vi "attribute_Express_SubVI.vi"(0 "VISA resource name":refnum<visa-resource-name>, 1 "Attribute ID":string, 2 "Attribute Operation":u16(ring)=1 items=["Read", "Write", "Read Direct", "Write Direct", "Write Fix", "Compose Direct", "Compose Fix"], 3 "SCPI Command":string, 4 "Direct cmd in":string, 5 "error in (no error)":errorcluster, 6 "Input I32":i32, 8 "Input Double":dbl format="%#_6p", 10 "Input String":string, 12 "Input Boolean":bool, 15 "Repeated Capabilities":string, 17 "Input I64":i64) -> (7 "Output I32":i32, 9 "Output Double":dbl, 11 "Output String":string, 13 "Output Boolean":bool, 14 "VISA resource name out":refnum<visa-resource-name>, 16 "Output I64":i64, 18 "Direct cmd out":string, 19 "error out":errorcluster)   [LabVIEW 2014, in "rszvl_rsidr_core.lvlib"]
uses:
  rszvl_rsidr_core.lvlib
  type_Attribute.ctl
  type_Attribute_Data_Type.ctl
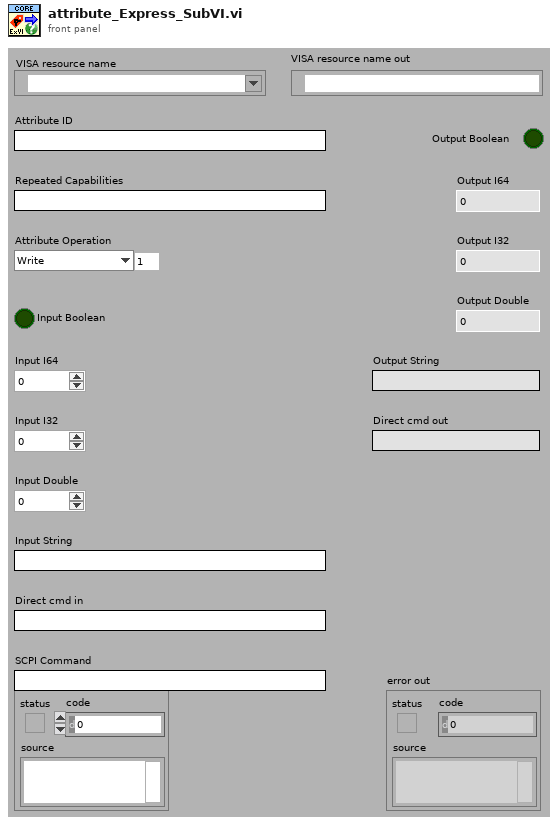
[diagram p1: front panel]
types:
  T1 = typedef "rszvl_rsidr_core.lvlib/type_Attribute.ctl" = cluster{"Identifier":string, "Descriptive name":string, "Data Type":T2, "Command":string, "Access":u16, "Range Table":string, "Read Callback":string, "Write Callback":string, "Range Callback":string, "Check Callback":string, "Rngtable Callback":string, "Coerce Callback":string, "Supported Models":string, "Instrument Options":string, "Repeated Capabilities":string, "Check Status Callback":string, "Index":i32, "Flag: OPC Wait":bool, "Flag: Dont check status":bool, "Flag: Cache Only":bool}
  T2 = typedef "rszvl_rsidr_core.lvlib/type_Attribute_Data_Type.ctl" = enum16{"Integer 32", "Double", "String", "Boolean", "None", "Integer 64"}
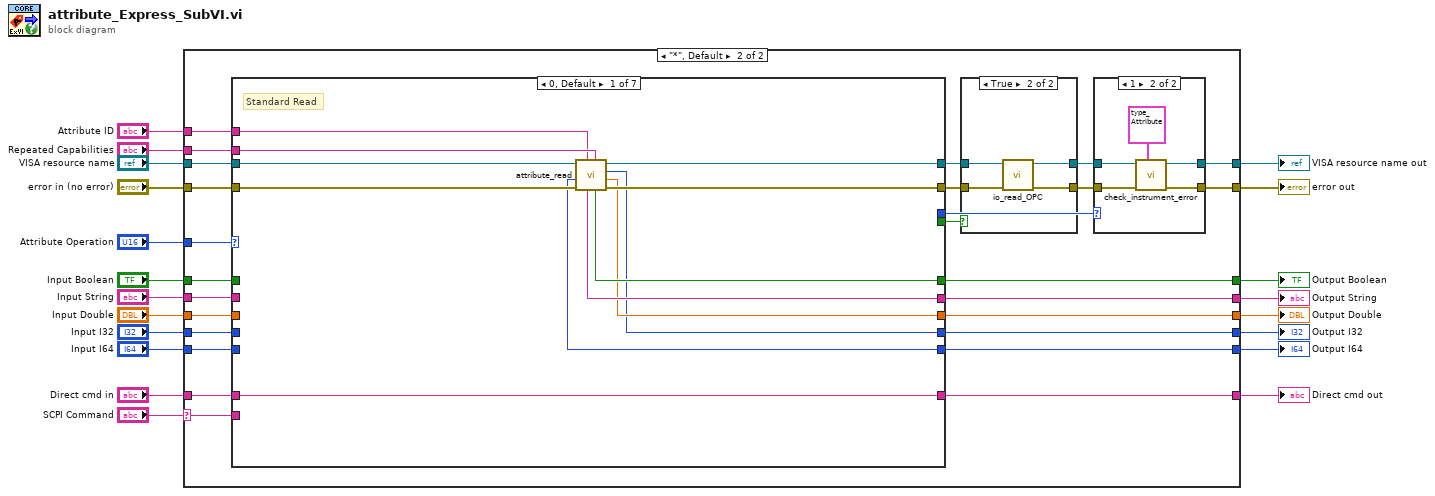
[diagram p0: block diagram]
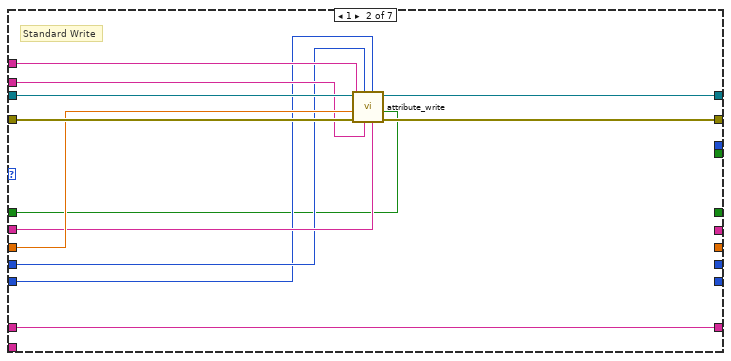
[diagram p5: hidden frame]
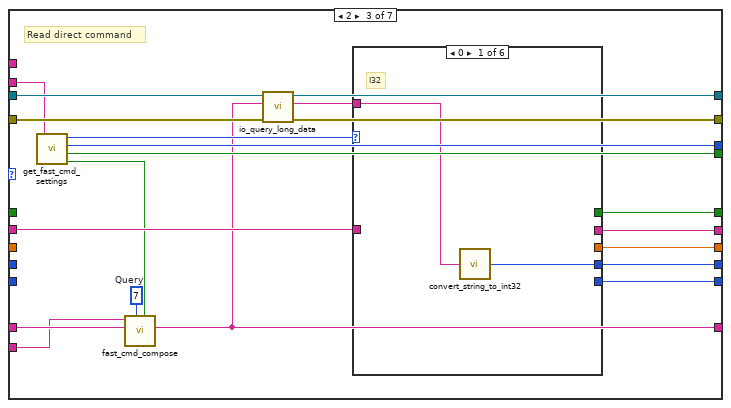
[diagram p6: hidden frame]
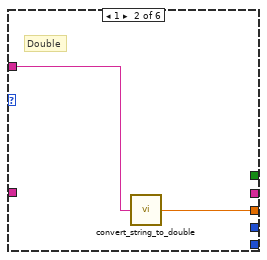
[diagram p7: hidden frame]
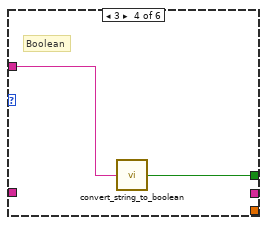
[diagram p9: hidden frame]
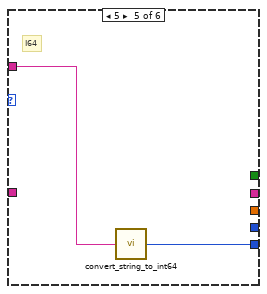
[diagram p10: hidden frame]
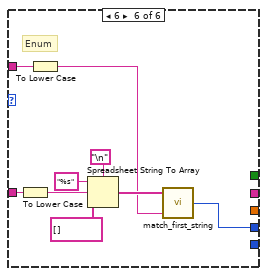
[diagram p11: hidden frame]
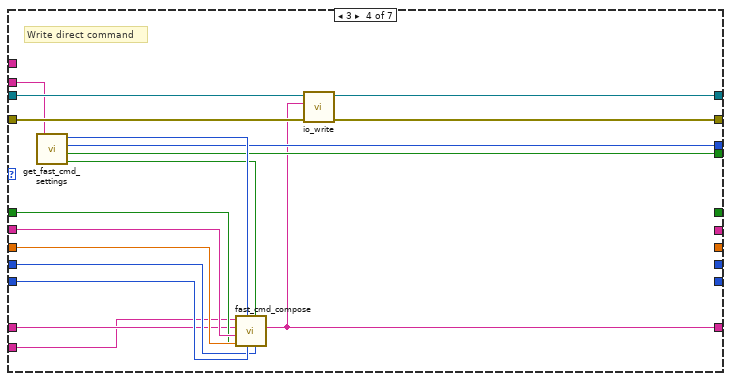
[diagram p12: hidden frame]
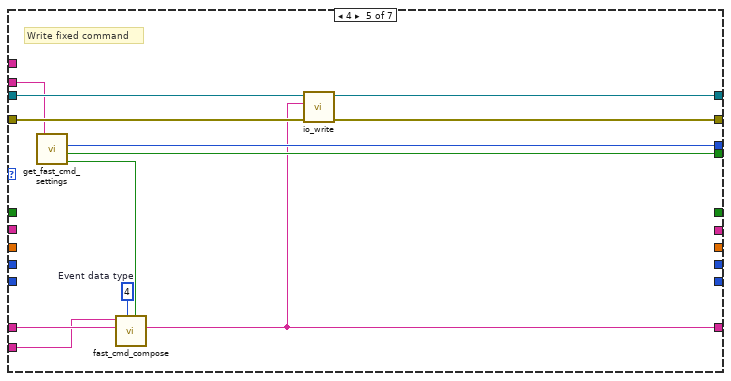
[diagram p13: hidden frame]
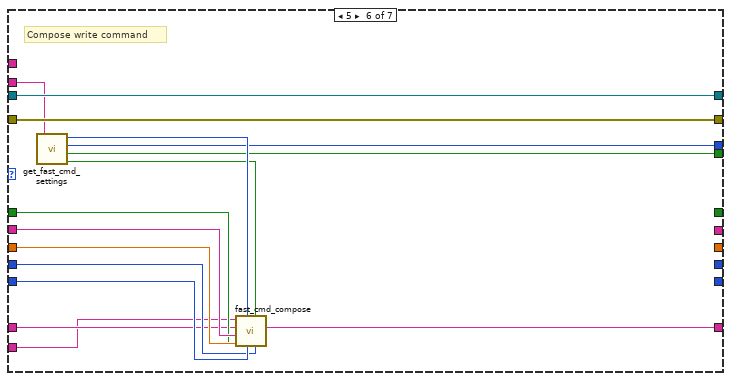
[diagram p14: hidden frame]
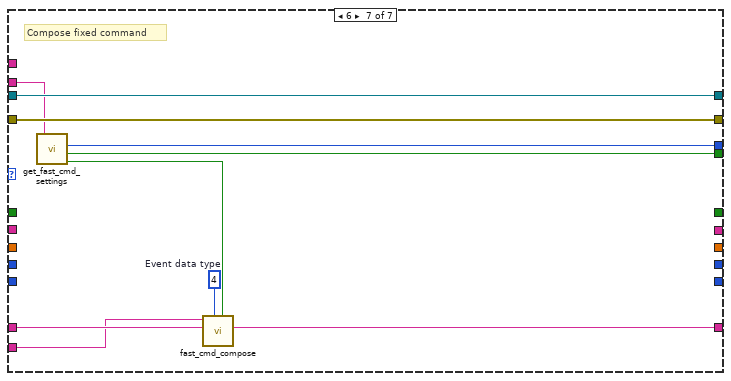
[diagram p15: hidden frame]
diagram:
  n1 = case shown="\"*\", Default" "SCPI Command" {
    selector: "SCPI Command" -> [_ w42]
    tunnel: "error in (no error)" -> [w27 w54]
    tunnel: "Direct cmd in" -> [w26 w53]
    tunnel: [w26 w52] -> w18
    tunnel: [w28 w45] -> w17
    tunnel: [w27 w44] -> w16
    tunnel: "VISA resource name" -> [w28 w43]
    tunnel: "Attribute Operation" -> [_ w41]
    tunnel: "Input Boolean" -> [w25 w40]
    tunnel: "Input String" -> [w24 w39]
    tunnel: "Input Double" -> [w23 w38]
    tunnel: "Input I32" -> [w22 w37]
    tunnel: "Input I64" -> [w21 w36]
    tunnel: [w25 w35] -> w8
    tunnel: [w24 w34] -> w7
    tunnel: [w23 w33] -> w6
    tunnel: [w22 w32] -> w5
    tunnel: [w21 w31] -> w4
    tunnel: "Repeated Capabilities" -> [_ w30]
    tunnel: "Attribute ID" -> [_ w29]
    frame "<skip>" {
    }
    frame "*", Default {
      n2 = case shown="0, Default" w41 {
        tunnel: w40 -> [_ w80 _ w144 _ w170 _]
        tunnel: w39 -> [_ w84 w104 w145 _ w171 _]
        tunnel: w38 -> [_ w85 _ w146 _ w172 _]
        tunnel: [w76 w88 w95 w133 w150 w173 w183] -> w49
        tunnel: [w77 w89 w94 w131 w149 w165 w180] -> w48
        tunnel: [w73 _ w107 _ _ _ _] -> w34
        tunnel: [w71 _ w108 _ _ _ _] -> w33
        tunnel: w43 -> [w75 w87 w97 w134 w151 w173 w183]
        tunnel: w54 -> [w78 w90 w98 w135 w152 w165 w180]
        tunnel: [w70 _ w109 _ _ _ _] -> w32
        tunnel: w37 -> [_ w82 _ w142 _ w168 _]
        tunnel: w36 -> [_ w81 _ w143 _ w169 _]
        tunnel: [w69 _ w110 _ _ _ _] -> w31
        tunnel: [w72 _ w106 _ _ _ _] -> w35
        tunnel: w53 -> [w79 w91 w111 w141 w158 w167 w182]
        tunnel: w42 -> [_ _ w101 w138 w155 w162 w177]
        tunnel: [w79 w91 w96 w132 w148 w166 w181] -> w52
        tunnel: [_ _ w103 w139 w156 w163 w178] -> w51
        tunnel: w30 -> [w74 w83 w92 w130 w147 w159 w174]
        tunnel: [_ _ w100 w137 w154 w161 w176] -> w50
        tunnel: w29 -> [w68 w86 _ _ _ _ _]
        frame 0, Default {
          # "Standard Read"
          n3 = call "attribute_read.vi"("Repeated Capability"=w74, "Attribute ID"=w68, "error in"=w78, "VISA resource name"=w75) -> ("error out"=w77:errorcluster, "Double out"=w71:dbl, "I32 out"=w70:i32, "VISA resource name out"=w76:refnum<visa-resource-name>, "Boolean out"=w72:bool, "String out"=w73:string, "I64 out"=w69:i64)  [unwired: 1 in]
        }
        frame 1 {
          # "Standard Write"
          n4 = call "attribute_write.vi"("Boolean in"=w80, "String in"=w84, "I64 in"=w81, "Repeated Capability"=w83, "I32 in"=w82, "error in"=w90, "Double in"=w85, "Attribute ID"=w86, "VISA resource name"=w87) -> ("error out"=w89:errorcluster, "VISA resource name out"=w88:refnum<visa-resource-name>)  [unwired: 1 in]
        }
        frame 2 {
          w105 = 7  # Query
          # "Read direct command"
          n5 = call "get_fast_cmd_settings.vi"("Settings in"=w92) -> ("*WAI"=w99:bool, "OPC?"=w100:bool, "ErrorCheckMode"=w103:i32, "DataType"=w102:i32)  [unwired: 3 in]
          n6 = call "fast_cmd_compose.vi"("*WAI (F)"=w99, "Data Type in"=w105, "Direct cmd in"=w111, "SCPI Command without parameter"=w101) -> ("Direct cmd out"=w96:string)  [unwired: 6 in, 1 out]
          n7 = call "io_query_long_data.vi"("error in"=w98, "write buffer"=w96, "VISA resource name"=w97) -> ("error out"=w94:errorcluster, "read buffer"=w93:string, "VISA resource name out"=w95:refnum<visa-resource-name>)  [unwired: 6 in]
          n8 = case shown="0" w102 {
            tunnel: w93 -> [w112 w114 w116 w118 w119 w125]
            tunnel: [_ _ _ _ w120 _] -> w110
            tunnel: [w113 _ _ _ _ w121] -> w109
            tunnel: [_ w115 _ _ _ _] -> w108
            tunnel: [_ _ w116 _ _ _] -> w107
            tunnel: [_ _ _ w117 _ _] -> w106
            tunnel: w104 -> [_ _ _ _ _ w129]
            frame 0 {
              # "I32"
              n9 = call "convert_string_to_int32.vi"("String in"=w112) -> ("int32 value out"=w113:i32)  [unwired: 4 in]
            }
            frame 1 {
              # "Double"
              n10 = call "convert_string_to_double.vi"("String in"=w114) -> ("double value out"=w115:dbl)  [unwired: 4 in]
            }
            frame 2, Default {
              # "String"
            }
            frame 3 {
              # "Boolean"
              n11 = call "convert_string_to_boolean.vi"("String in"=w118) -> ("boolean value out"=w117:bool)  [unwired: 4 in]
            }
            frame 5 {
              # "I64"
              n12 = call "convert_string_to_int64.vi"("String in"=w119) -> ("int64 value out"=w120:i64)  [unwired: 4 in]
            }
            frame 6 {
              # "Enum"
              n13 = To Lower Case(string=w129) -> (all lower case string=w124:string)
              n14 = To Lower Case(string=w125) -> (all lower case string=w122:string)
              n15 = Spreadsheet String To Array(delimiter (Tab)="\n" ("Line Feed Constant"), format string="%s", spreadsheet string=w124, array type (2D Dbl)=string[] []) -> (array=w123:string[])
              n16 = call "match_first_string.vi"("String to match"=w122, "Array in"=w123) -> ("Index out"=w121:i32)  [unwired: 3 in]
            }
          }
        }
        frame 3 {
          # "Write direct command"
          n17 = call "get_fast_cmd_settings.vi"("Settings in"=w130) -> ("*WAI"=w136:bool, "OPC?"=w137:bool, "ErrorCheckMode"=w139:i32, "DataType"=w140:i32)  [unwired: 3 in]
          n18 = call "fast_cmd_compose.vi"("Input Double (0.0)"=w146, "Input I32 (0)"=w142, "*WAI (F)"=w136, "Input I64 (0)"=w143, "Data Type in"=w140, "Input Boolean (F)"=w144, "Input String (\"\")"=w145, "Direct cmd in"=w141, "SCPI Command without parameter"=w138) -> ("Direct cmd out"=w132:string)  [unwired: 1 in, 1 out]
          n19 = call "io_write.vi"("error in"=w135, "write buffer"=w132, "VISA resource name"=w134) -> ("error out"=w131:errorcluster, "VISA resource name out"=w133:refnum<visa-resource-name>)  [unwired: 7 in]
        }
        frame 4 {
          w157 = 4  # Event data type
          # "Write fixed command"
          n20 = call "get_fast_cmd_settings.vi"("Settings in"=w147) -> ("*WAI"=w153:bool, "OPC?"=w154:bool, "ErrorCheckMode"=w156:i32)  [unwired: 3 in, 1 out]
          n21 = call "fast_cmd_compose.vi"("*WAI (F)"=w153, "Data Type in"=w157, "Direct cmd in"=w158, "SCPI Command without parameter"=w155) -> ("Direct cmd out"=w148:string)  [unwired: 6 in, 1 out]
          n22 = call "io_write.vi"("error in"=w152, "write buffer"=w148, "VISA resource name"=w151) -> ("error out"=w149:errorcluster, "VISA resource name out"=w150:refnum<visa-resource-name>)  [unwired: 7 in]
        }
        frame 5 {
          # "Compose write command"
          n23 = call "get_fast_cmd_settings.vi"("Settings in"=w159) -> ("*WAI"=w160:bool, "OPC?"=w161:bool, "ErrorCheckMode"=w163:i32, "DataType"=w164:i32)  [unwired: 3 in]
          n24 = call "fast_cmd_compose.vi"("Input Double (0.0)"=w172, "Input I32 (0)"=w168, "*WAI (F)"=w160, "Input I64 (0)"=w169, "Data Type in"=w164, "Input Boolean (F)"=w170, "Input String (\"\")"=w171, "Direct cmd in"=w167, "SCPI Command without parameter"=w162) -> ("Direct cmd out"=w166:string)  [unwired: 1 in, 1 out]
        }
        frame 6 {
          w179 = 4  # Event data type
          # "Compose fixed command"
          n25 = call "get_fast_cmd_settings.vi"("Settings in"=w174) -> ("*WAI"=w175:bool, "OPC?"=w176:bool, "ErrorCheckMode"=w178:i32)  [unwired: 3 in, 1 out]
          n26 = call "fast_cmd_compose.vi"("*WAI (F)"=w175, "Data Type in"=w179, "Direct cmd in"=w182, "SCPI Command without parameter"=w177) -> ("Direct cmd out"=w181:string)  [unwired: 6 in, 1 out]
        }
      }
      n27 = case shown="True" w50 {
        tunnel: w48 -> [w55 w60]
        tunnel: [w55 w58] -> w46
        tunnel: [w56 w57] -> w47
        tunnel: w49 -> [w56 w59]
        frame False {
        }
        frame True {
          n28 = call "io_read_OPC.vi"("error in"=w60, "VISA resource name"=w59) -> ("error out"=w58:errorcluster, "VISA resource name out"=w57:refnum<visa-resource-name>)  [unwired: 7 in, 1 out]
        }
      }
      n29 = case shown="1" w51 {
        tunnel: w46 -> [w61 w67]
        tunnel: [w61 w65] -> w44
        tunnel: [w62 w64] -> w45
        tunnel: w47 -> [w62 w66]
        frame 0, Default {
        }
        frame 1 {
          n30 = call "check_instrument_error.vi"("Attribute"=T1 {"Identifier"="", "Descriptive name"="", "Data Type"=enum."Integer 32", "Command"="", "Access"=2, "Range Table"="", "Read Callback"="", "Write Callback"="", "Range Callback"="", "Check Callback"="", "Rngtable Callback"="", "Coerce Callback"="", "Supported Models"="", "Instrument Options"="", "Repeated Capabilities"="", "Check Status Callback"="", "Index"=0, "Flag: OPC Wait"=FALSE, "Flag: Dont check status"=FALSE, "Flag: Cache Only"=FALSE}, "error in"=w67, "VISA resource name"=w66) -> ("error out"=w65:errorcluster, "VISA resource name out"=w64:refnum<visa-resource-name>)  [unwired: 7 in]
        }
      }
    }
  }
  "error out" <- w16
  "VISA resource name out" <- w17
  "Direct cmd out" <- w18
  "Output I64" <- w4
  "Output Double" <- w6
  "Output String" <- w7
  "Output Boolean" <- w8
  "Output I32" <- w5
